vi "modify.vi"(8 "error in (no error)":errorcluster, 11 "GenericStringGenerator in":refnum<class "GenericStringGenerator.lvclass">) -> (0 "error out":errorcluster, 2 "String":string, 3 "GenericStringGenerator out":refnum<class "GenericStringGenerator.lvclass">)   [LabVIEW 2010, in "GenericStringGenerator.lvclass"]
uses:
  GenericStringGenerator.lvclass
panel:
  # "This functionality is not implemented for this component \n(i.e., for GenericStringGenerator)."
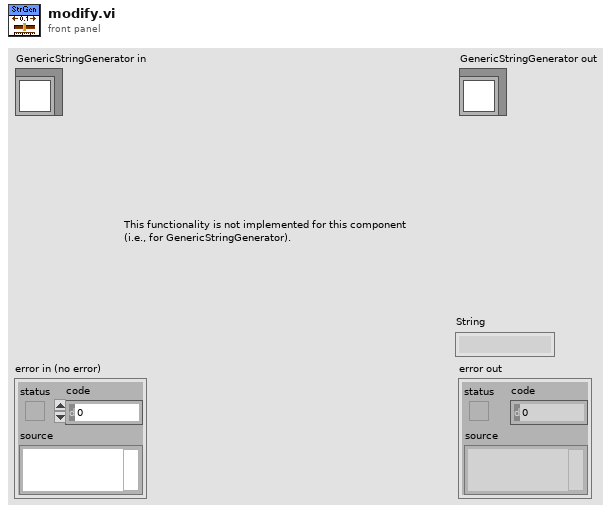
[diagram p1: front panel]
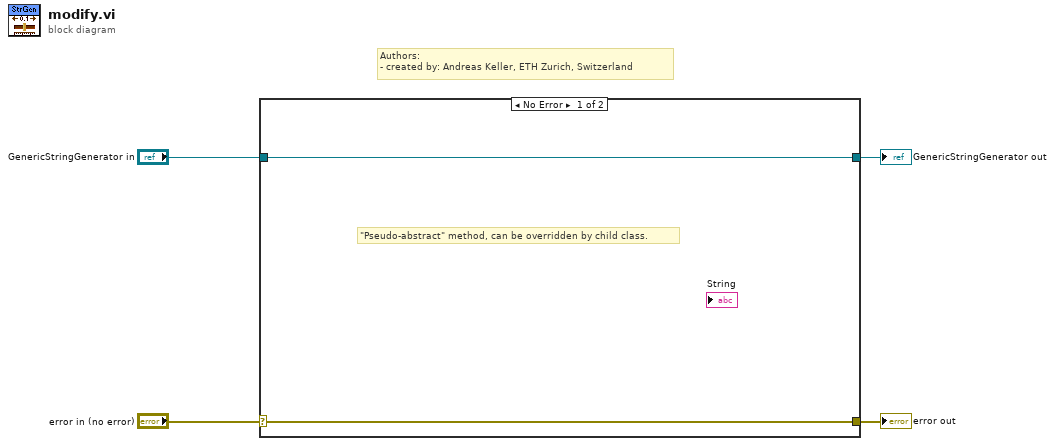
[diagram p0: block diagram]
diagram:
  # "Authors: \n- created by: Andreas Keller, ETH Zurich, Switzerland"
  n1 = case shown="No Error" "error in (no error)" {
    selector: "error in (no error)" -> [w5 w8]
    tunnel: [w5 w8] -> w3
    tunnel: [w6 w7] -> w1
    tunnel: "GenericStringGenerator in" -> [w6 w7]
    frame No Error {
      # "\"Pseudo-abstract\" method, can be overridden by child class."
    }
    frame Error {
    }
  }
  "error out" <- w3
  "GenericStringGenerator out" <- w1
